vi "sine.vi"() -> ()   [LabVIEW 2021]
uses:
  <vilib>/express/express analysis/Spectral/Block/exnSpectralBlock spectral measurements power poly.vi
  <vilib>/express/express analysis/Spectral/Block/exnSpectralBlock spectral measurements power WFM.vi
  <vilib>/express/express analysis/Spectral/XNode/ExpressSpectralMeasurementsBlockNode.xnode
  <vilib>/Analysis/NI_AALBase.lvlib
panel:
  out "Waveform Graph 2":cluster{"f0":dbl, "df":dbl, "magnitude":dbl[]}(graph)
  out "Waveform Graph":dbl[](graph)
  out "Numeric":dbl
  out "Array":dbl[](array[numeric])
  out "sine wave":dbl[][](array[numeric])
  in  "sampling rate":dbl
  in  "v":dbl
  in  "path diff":dbl
  in  "wavenumber":dbl[](array[numeric])
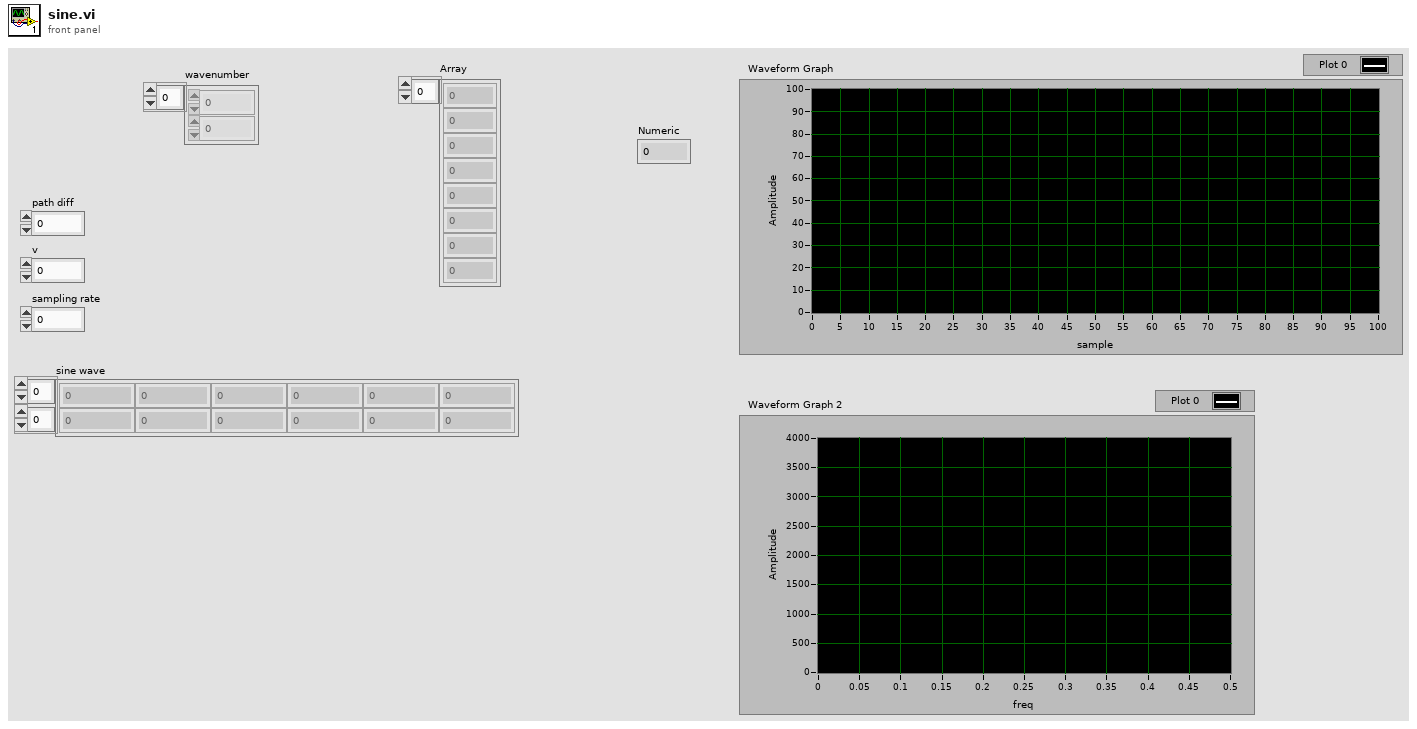
[diagram p1: front panel]
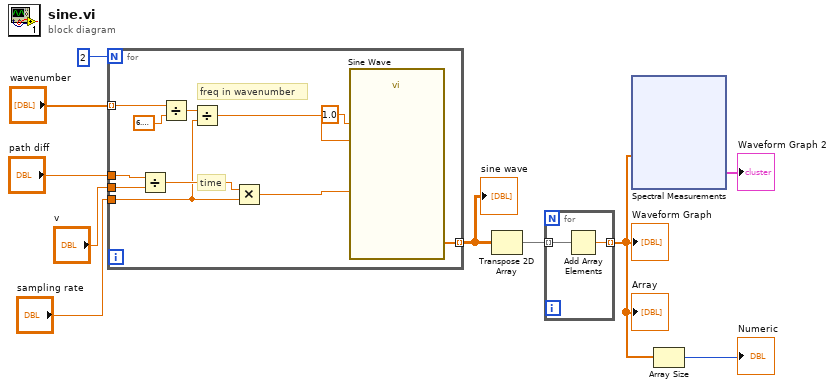
[diagram p0: block diagram]
diagram:
  n1 = for {
    N: 2 -> [_]
    tunnel: "wavenumber" -> [w20] mode=indexing
    tunnel: "path diff" -> [w19]
    tunnel: "v" -> [w18]
    tunnel: "sampling rate" -> [w13]
    tunnel: [w16] -> w6 mode=indexing
    # "time"
    # "freq in wavenumber"
    n2 = Divide(x=w19, y=w18) -> (x/y=w17:dbl)
    n3 = Divide(x=w20, y=6.283185307179586) -> (x/y=w14:dbl)
    n4 = Divide(x=w14, y=w13) -> (x/y=w12:dbl)
    n5 = Multiply(x=w17, y=w13) -> (x*y=w15:dbl)
    n6 = call <vilib>:"Sine Wave.vi"("samples"=w15, "amplitude"=1.0, "frequency"=w12) -> ("sine wave"=w16:dbl[])  [unwired: 2 in, 2 out]
  }
  "sine wave" <- w6
  n7 = Transpose 2D Array(2D array=w6) -> (transposed array=w5:dbl[][])
  n8 = for {
    tunnel: w5 -> [w23] mode=indexing
    tunnel: [w22] -> w3 mode=indexing
    n9 = Add Array Elements(numeric array=w23) -> (sum=w22:dbl)
  }
  "Array" <- w3
  "Waveform Graph" <- w3
  n10 = xnode "Spectral Measurements"("Signals"=w3) -> ("Power Spectrum"=→"Waveform Graph 2":cluster{"f0":dbl, "df":dbl, "magnitude":dbl[]})  [unwired: 1 in, 1 out]
  n11 = Array Size(array=w3) -> (size(s)=→"Numeric":i32)
